vi "Query RF Connection Direction.vi"(8 "error in (no error)":errorcluster, 10 "RF Connection (\"RF1.1\")":string="RF1.1", 11 "VISA resource name":refnum<visa-resource-name>) -> (0 "error out":errorcluster, 3 "VISA resource name out":refnum<visa-resource-name>)   [LabVIEW 2015, in "Rohde&Schwarz CMXP Base.lvlib"]
doc: "Queries the direction of a signal path (TX/RX of the instrument).\n\nAttribute:\n-\n\nRemote-control command:\n[CONFigure:]TENVironment:SPATh:DIRection?"
uses:
  <instrlib>/Rohde&Schwarz CMXP Base/Rohde&Schwarz CMXP Base.lvlib
  <instrlib>/Rohde&Schwarz CMXP Base/Private/rsidr_core.llb/rsidr_core.lvlib
panel:
  out "Direction":i32(ring) items=["", "TX", "TX & RX"]
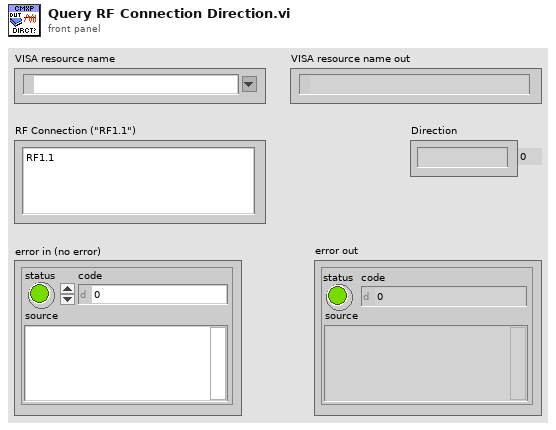
[diagram p1: front panel]
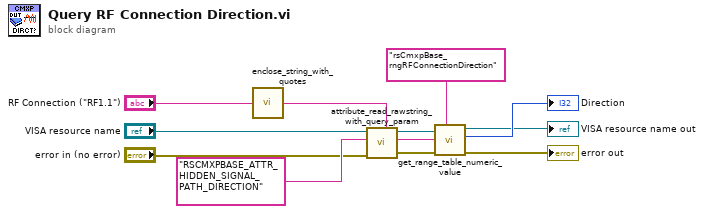
[diagram p0: block diagram]
diagram:
  n1 = call <instrlib>:"enclose_string_with_quotes.vi"("String to enclose"="RF Connection (\"RF1.1\")") -> ("String out"=w1:string)  [unwired: 4 in]
  n2 = call <instrlib>:"attribute_read_rawstring_with_query_param.vi"("Query Parameter (None)"=w1, "error in"="error in (no error)", "Attribute ID"="RSCMXPBASE_ATTR_HIDDEN_SIGNAL_PATH_DIRECTION", "VISA resource name"="VISA resource name") -> ("error out"=w11:errorcluster, "RawString out"=w10:string, "VISA resource name out"=w12:refnum<visa-resource-name>)  [unwired: 5 in]
  n3 = call <instrlib>:"get_range_table_numeric_value.vi"("Range Table ID in"="rsCmxpBase_rngRFConnectionDirection", "error in"=w11, "String Value"=w10, "VISA resource name"=w12) -> ("error out"=→"error out":errorcluster, "I32 output"=→"Direction":i32, "VISA resource name out"=→"VISA resource name out":refnum<visa-resource-name>)  [unwired: 5 in]
